vi "delete dataset.vi"(7 "existing file numbers":string[](array[string]), 8 "existing data cluster":cluster{"array type (2D Dbl)":dbl[][]}[](array[cluster])) -> (1 "survived dataset names":string[](array[string]), 2 "survived dataset":cluster{"array type (2D Dbl)":dbl[][]}[](array[cluster]))   [LabVIEW 2019]
panel:
  in  "Done?":bool
  in  "Dara Sets (check box to delete)":cluster{string, bool}[](array[cluster])
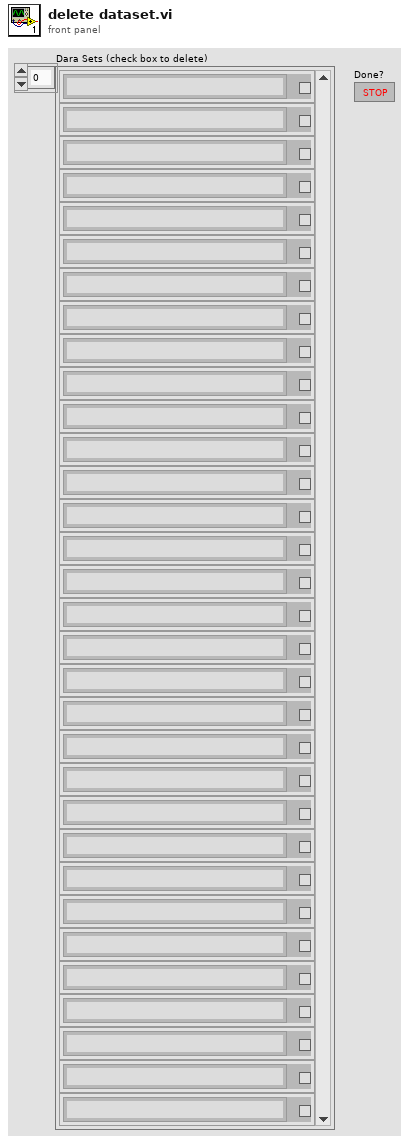
[diagram p1: front panel]
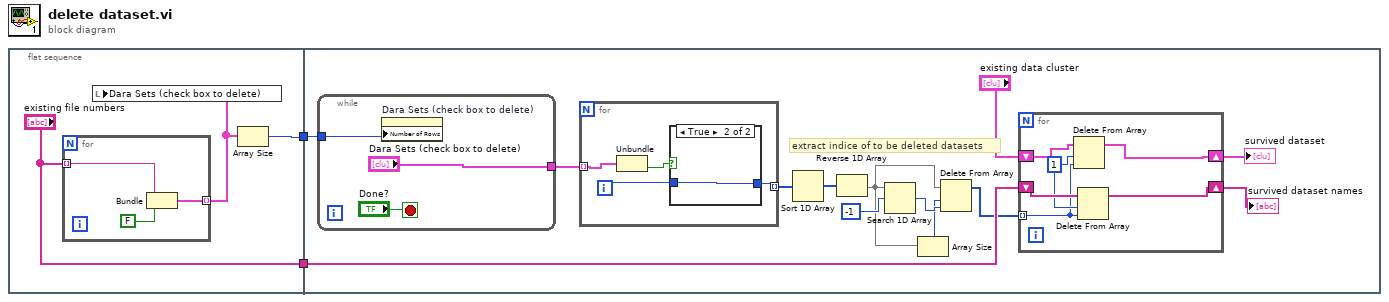
[diagram p0: block diagram]
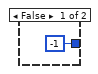
[diagram p2: hidden frame]
diagram:
  n1 = flat-sequence {
    tunnel: [w4] -> w2
    tunnel: ["existing file numbers"] -> w1
    tunnel: w2 -> [w21]
    tunnel: w1 -> [w12]
    frame #0 {
      n2 = for {
        tunnel: "existing file numbers" -> [w8] mode=indexing
        tunnel: [w6] -> w5 mode=indexing
        n3 = Bundle(w8, FALSE) -> (w6:cluster{string, bool})  [unwired: 1 in]
      }
      n4 = local write "Dara Sets (check box to delete)"(w5) -> ()
      n5 = Array Size(array=w5) -> (size(s)=w4:i32)
    }
    frame #1 {
      # "extract indice of to be deleted datasets"
      n6 = while {
        tunnel: w21 -> [w35]
        tunnel: ["Dara Sets (check box to delete)"] -> w20
        stop <- "Done?" stop-if-true
        n7 = property on="Dara Sets (check box to delete)" class="Arr (strict)"("Number of Rows"=w35) -> ()  [unwired: 2 in, 2 out]
      }
      n8 = for {
        tunnel: w20 -> [w31] mode=indexing
        tunnel: [w28] -> w19 mode=indexing
        i -> [w29]
        n9 = Unbundle(w31) -> (w30:bool)  [unwired: 1 out]
        n10 = case shown="True" w30 {
          tunnel: w29 -> [_ w33]
          tunnel: [-1 w33] -> w28
          frame False {
          }
          frame True {
          }
        }
      }
      n11 = Sort 1D Array(array=w19) -> (sorted array=w18:i32[])
      n12 = Reverse 1D Array(array=w18) -> (reversed array=w15:i32[])
      n13 = Search 1D Array(1D array=w15, element=-1) -> (index of element=w16:i32)  [unwired: 1 in]
      n14 = Array Size(array=w15) -> (size(s)=w14:i32)
      n15 = Delete From Array(array=w15, length=w14, index=w16) -> (array with subset deleted=w11:i32[])  [unwired: 1 out]
      n16 = for {
        shift-right: [w23] -> w10
        shift-left: "existing data cluster" -> [w27]
        shift-right: [w22] -> w9
        shift-left: w12 -> [w26]
        tunnel: w11 -> [w24] mode=indexing
        w25 = 1 ("length")
        n17 = Delete From Array(array=w27, length=w25, index=w24) -> (array with subset deleted=w23:cluster{"array type (2D Dbl)":dbl[][]}[])  [unwired: 1 out]
        n18 = Delete From Array(array=w26, length=w25, index=w24) -> (array with subset deleted=w22:string[])  [unwired: 1 out]
      }
      "survived dataset" <- w10
      "survived dataset names" <- w9
    }
  }
